vi "Average Waveform.vi"(11 "Channel in":waveform(dbl)={"t0"=timestamp(0 s since 1904-01-01), "dt"=1.0, "Y"=[1.0]}) -> (2 "Quiescent":dbl, 3 "Channel Out":waveform(dbl)={"t0"=timestamp(0 s since 1904-01-01), "dt"=1.0, "Y"=[1.0]})   [LabVIEW 2019, in "Variant Parser.lvlib" / "Variant Parser.lvclass"]
uses:
  Library/Variant Parser.lvclass
  <vilib>/Analysis/baseanly.llb/Mean (DBL).vi
  <vilib>/Analysis/NI_AALBase.lvlib
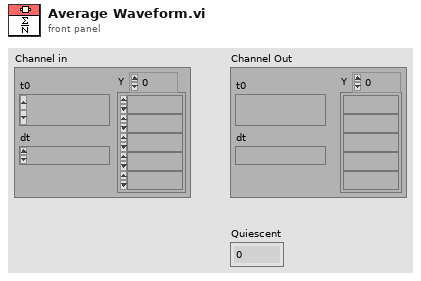
[diagram p1: front panel]
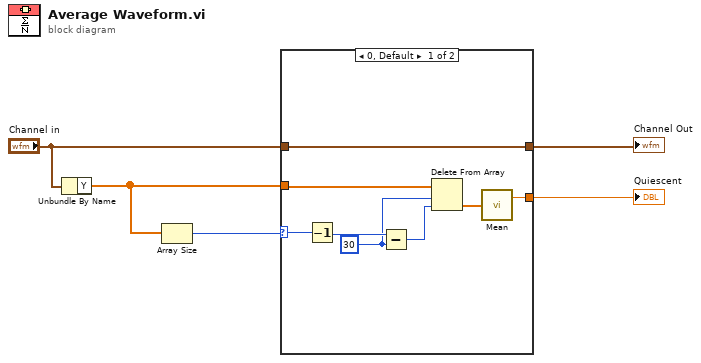
[diagram p0: block diagram]
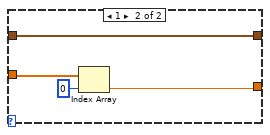
[diagram p2: hidden frame]
diagram:
  n1 = Unbundle By Name("Channel in") -> ("Y"=w2:dbl[])
  n2 = Array Size(array=w2) -> (size(s)=w5:i32)
  n3 = case shown="0, Default" w5 {
    selector: w5 -> [w6 _]
    tunnel: "Channel in" -> [w13 w17]
    tunnel: [w13 w17] -> w3
    tunnel: w2 -> [w8 w16]
    tunnel: [w7 w15] -> w1
    frame 0, Default {
      w10 = 30 ("y")
      n4 = Decrement(x=w6) -> (x-1=w12:i32)
      n5 = Subtract(x=w12, y=w10) -> (x-y=w11:i32)
      n6 = Delete From Array(array=w8, length=w10, index=w11) -> (deleted portion=w9:dbl[])  [unwired: 1 out]
      n7 = call-poly <vilib>:"Mean.vi"("X"=w9) -> ("mean"=w7:dbl)  [unwired: 1 out]
    }
    frame 1 {
      n8 = Index Array(array=w16, index=0) -> (element=w15:dbl)
    }
  }
  "Channel Out" <- w3
  "Quiescent" <- w1
